vi "Axe In Range.vi"(1 "RangeNumber":dbl, 2 "Axe":dbl) -> (0 "NumericGlobalData":dbl)   [LabVIEW 2018]
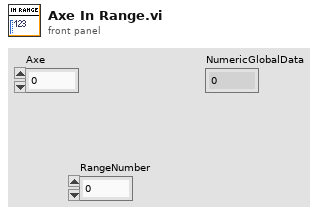
[diagram p1: front panel]
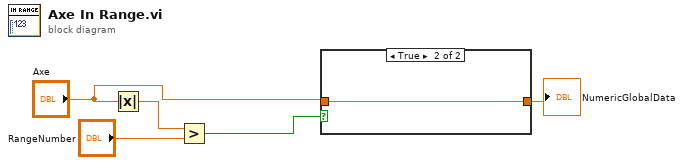
[diagram p0: block diagram]
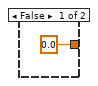
[diagram p2: hidden frame]
diagram:
  n1 = Absolute Value(x="Axe") -> (abs(x)=w5:dbl)
  n2 = Greater?(x=w5, y="RangeNumber") -> (0:w4:bool)
  n3 = case shown="True" w4 {
    tunnel: "Axe" -> [_ w7]
    tunnel: [0.0 ("Numeric") w7] -> w3
    frame False {
    }
    frame True {
    }
  }
  "NumericGlobalData" <- w3
